vi "Remove Empty Lines from String.vi"(11 "String":string) -> (3 "String Out":string)   [LabVIEW 2016, in "SLL String.lvlib"]
doc: "Removes empty lines present in the multi line string."
uses:
  SLL String.lvlib
  _SubVIs/String to 1D String Array.vi
  _SubVIs/1D String Array to String.vi
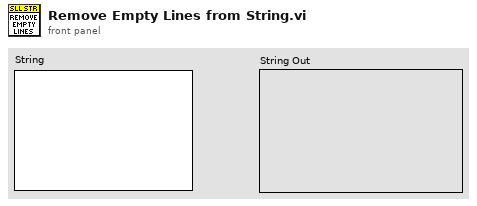
[diagram p1: front panel]
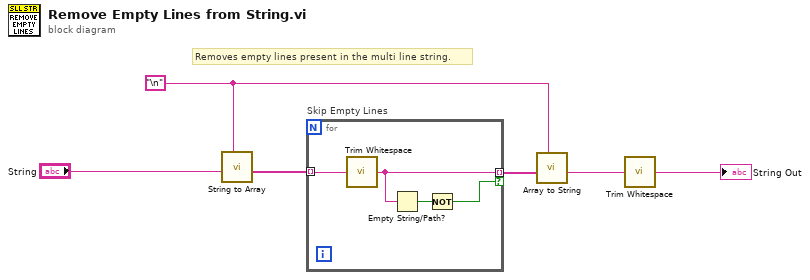
[diagram p0: block diagram]
diagram:
  w3 = "\n"
  # "Removes empty lines present in the multi line string."
  n1 = call-poly "String to Array.vi"("Delimiter (,)"=w3, "String"="String") -> ("Array[]"=w5:string[])  [unwired: 6 in]
  n2 = for "Skip Empty Lines" {
    tunnel: w5 -> [w10] mode=indexing
    tunnel: [w9] -> w4 mode=indexing if=w7
    n3 = call <vilib>:"Trim Whitespace.vi"("string"=w10) -> ("trimmed string"=w9:string)  [unwired: 1 in]
    n4 = Empty String/Path?(string/path=w9) -> (empty?=w8:bool)
    n5 = Not(x=w8) -> (.not. x?=w7:bool)
  }
  n6 = call-poly "Array to String.vi"("Delimiter (,)"=w3, "1D Array[]"=w4) -> ("String"=w2:string)  [unwired: 6 in]
  n7 = call <vilib>:"Trim Whitespace.vi"("string"=w2) -> ("trimmed string"=→"String Out":string)  [unwired: 1 in]
